vi "ReadSignalFromTXT_TU.vi"() -> ()   [LabVIEW 2025]
panel:
  out "signal out":waveform(dbl)(graph)
  out "error out":errorcluster
  in  "file path in":path
  in  "error in":errorcluster
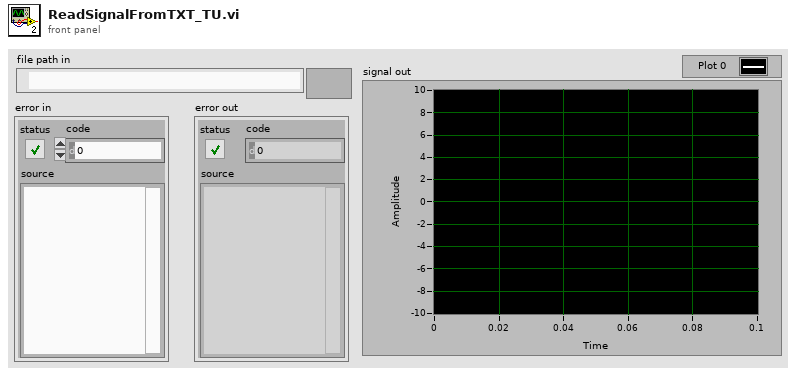
[diagram p1: front panel]
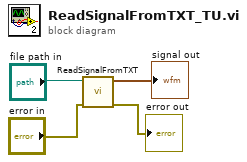
[diagram p0: block diagram]
diagram:
  n1 = call "ReadSignalFromTXT.vi"("error in"="error in", "file path in"="file path in") -> ("error out"=→"error out":errorcluster, "signal out"=→"signal out":waveform(dbl))  [unwired: 8 in]
